vi "Close.vi"(5 "Close I2C Master?":bool, 7 "I2C Channel (0)":u8, 8 "Error In":errorcluster, 10 "I2C Slave Address":T1, 11 "LINX Resource":T2) -> (0 "Error Out":errorcluster, 3 "LINX Resource":T2)   [LabVIEW 2014, in "LMH-LINX.lvlib" / "ADXL345.lvlib"]
doc: "Close the ADXL345 and optionally close the I2C master."
uses:
  <vilib>/MakerHub/LINX/Public/Sensors/Accelerometer/ADXL345/ADXL345.lvlib
  <vilib>/MakerHub/LINX/Private/Type Defs/LINX Ref.ctl
  <vilib>/MakerHub/LINX/Private/Type Defs/Platform.ctl
  <vilib>/MakerHub/LINX/Private/Type Defs/Interface.ctl
  <vilib>/MakerHub/LINX/Private/Device/Type Defs/LINX Device Config.ctl
  <vilib>/MakerHub/LINX/Private/Device/Type Defs/TCP Config.ctl
  <vilib>/MakerHub/LINX/Private/Device/Type Defs/Channels.ctl
  <vilib>/MakerHub/LINX/Public/Sensors/Accelerometer/ADXL345/Address.ctl
  <vilib>/MakerHub/LINX/LMH-LINX.lvlib
  <vilib>/MakerHub/LINX/Private/Device/Device.lvlib
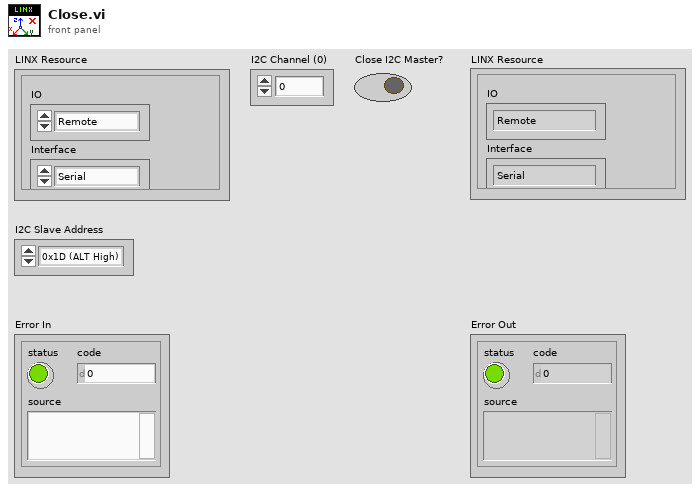
[diagram p1: front panel]
types:
  T1 = typedef "LMH-LINX.lvlib/ADXL345.lvlib/Address.ctl" = enum16{"0x1D (ALT High)", "0x53 (ALT Low)"}
  T2 = typedef "LMH-LINX.lvlib/LINX Ref.ctl" = cluster{"IO":T3, "Interface":T4, "LINX Device Config":T5}
  T3 = typedef "LMH-LINX.lvlib/Platform.ctl" = enum16{"Remote", "Local"}
  T4 = typedef "LMH-LINX.lvlib/Interface.ctl" = enum16{"Serial", "TCP"}
  T5 = typedef "LMH-LINX.lvlib/Device.lvlib/LINX Device Config.ctl" = cluster{"Interface":T4, "COM Port":refnum<visa-resource-name>, "TCP Configuration":T6, "Device Family":u8, "Device ID":u8, "Device Name":string, "TCP Ref":refnum<k5>, "Channels":T7}
  T6 = typedef "LMH-LINX.lvlib/Device.lvlib/TCP Config.ctl" = cluster{"IP Address":string, "Port":u16}
  T7 = typedef "LMH-LINX.lvlib/Channels.ctl" = cluster{"DI":u8[], "DO":u8[], "AI":u8[], "AO":u8[], "PWM":u8[], "QE":u8[], "UART":u8[], "I2C 2":u8[], "SPI":u8[], "CAN":u8[], "Servo":u8[], "AI Ref (V)":dbl, "AI Resolution (Bits)":u8, "AO Ref (V)":dbl, "AO Resolution (Bits)":u8}
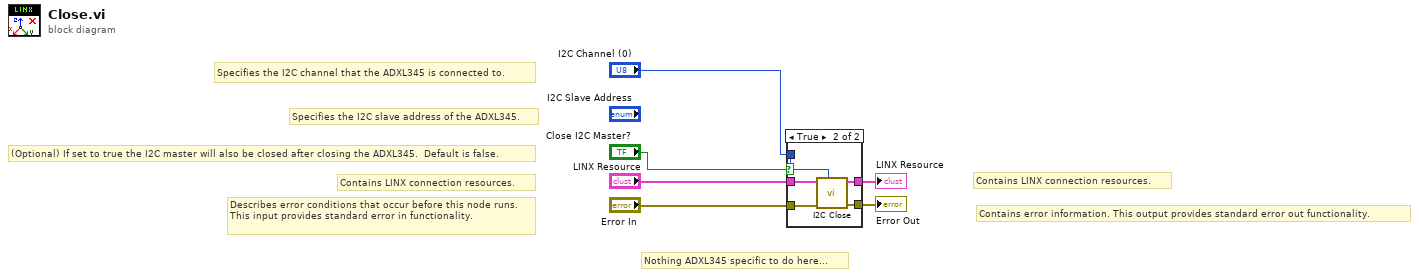
[diagram p0: block diagram]
diagram:
  # "Specifies the I2C slave address of the ADXL345."
  # "Specifies the I2C channel that the ADXL345 is connected to."
  # "(Optional) If set to true the I2C master will also be closed after closing the ADXL345.  Default is false."
  # "Contains LINX connection resources."
  # "Contains error information. This output provides standard error out functionality."
  # "Contains LINX connection resources."
  # "Describes error conditions that occur before this node runs. This input provides standard error in functionality."
  # "Nothing ADXL345 specific to do here..."
  n1 = case shown="True" "Close I2C Master?" {
    tunnel: "Error In" -> [w7 w13]
    tunnel: "LINX Resource" -> [w8 w12]
    tunnel: [w8 w11] -> w4
    tunnel: [w7 w10] -> w3
    tunnel: "I2C Channel (0)" -> [_ w9]
    frame False {
    }
    frame True {
      n2 = call <vilib>:"I2C Close.vi"("I2C Channel (0)"=w9, "Error In"=w13, "LINX Resource"=w12) -> ("Error Out"=w10:errorcluster, "LINX Resource"=w11:T2)  [unwired: 7 in]
    }
  }
  "LINX Resource" <- w4
  "Error Out" <- w3
